vi "LatchButton.vi"(11 "Boolean In":bool=TRUE) -> (3 "Boolean Out":bool)   [LabVIEW 2019]
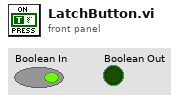
[diagram p1: front panel]
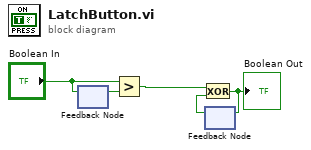
[diagram p0: block diagram]
diagram:
  n1 = feedback #1() -> (w1:bool)  [unwired: 1 in]
  n2 = feedback-in #1("Boolean In") -> ()
  n3 = Greater?(x="Boolean In", y=w1) -> (0:w3:bool)
  n4 = feedback #2() -> (w4:bool)  [unwired: 1 in]
  n5 = Exclusive Or(1:w4, 2:w3) -> (0:w5:bool)
  "Boolean Out" <- w5
  n6 = feedback-in #2(w5) -> ()
